vi "_FG_save_data.vi"(0 "enum":T1=enum."write", 2 "filenames (array)":string[](array[string]), 5 "entete":string, 7 "data in":variant, 9 "end":string, 11 "error in":errorcluster, 12 "array in line ?":bool, 13 "indexes to write":i32[](array[numeric])) -> (4 "path Array":path[](array[path]), 15 "error out":errorcluster)   [LabVIEW 2019]
uses:
  ae_save_data.ctl
  <userlib>/_OpenG.lib/array/array.llb/Index 1D Array Elements (Path)__ogtk.vi
  <vilib>/Utility/Data Type/NI_Data Type.lvlib
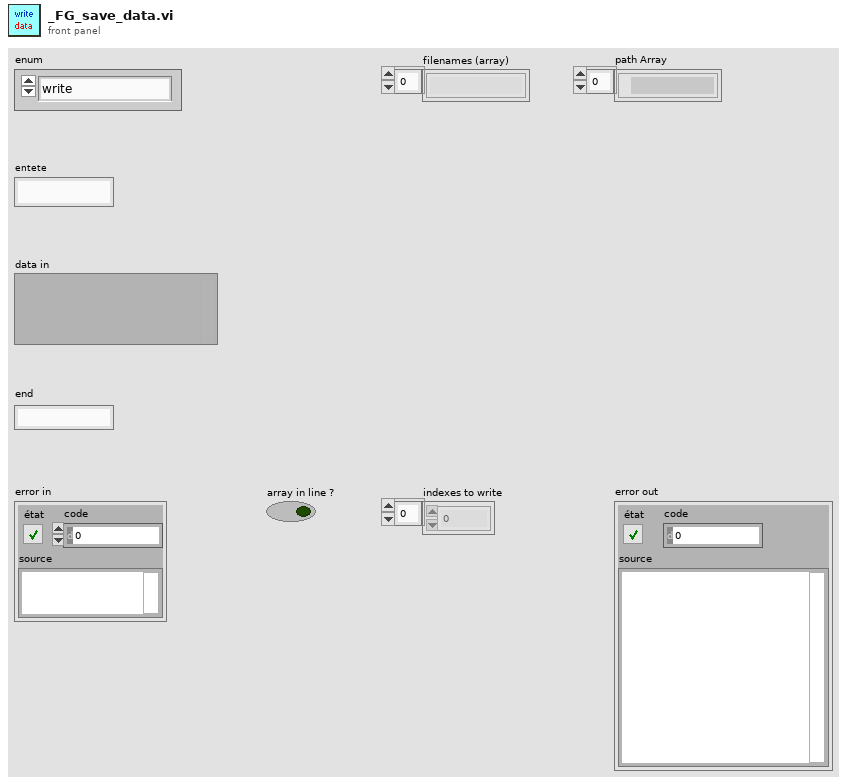
[diagram p1: front panel]
types:
  T1 = typedef "ae_save_data.ctl" = enum16{"create_file", "write", "time", "close_file", "read"}
  T2 = enum16{"open", "replace", "create", "open or create", "replace or create", "replace or create with confirmation"}
  T3 = typedef "NI_Data Type.lvlib/Data Type.ctl" = enum8{"Invalid Type", "Void", "I8", "I16", "I32", "I64", "U8", "U16", "U32", "U64", "Single Float", "Double Float", "Extended Float", "Single Complex", "Double Complex", "Extended Complex", "Enum U8", "Enum U16", "Enum U32", "Enum U64", "Single Float With Unit", "Double Float With Unit", "Extended Float With Unit", "Single Complex with Unit", "Double Complex with Unit", "Extended Complex with Unit", "Boolean", "String", "Path", "Picture", "Tag", "Array", "Cluster", "Variant", "LV Variant", "Waveform", "Timestamp", "Digital Waveform", "Digital Data", "ExpressData", "Refnum", "External Data", "VI", "Poly VI", "LabVIEW Class Instance", "Fixed Point", "Set Collection", "Map Collection"}
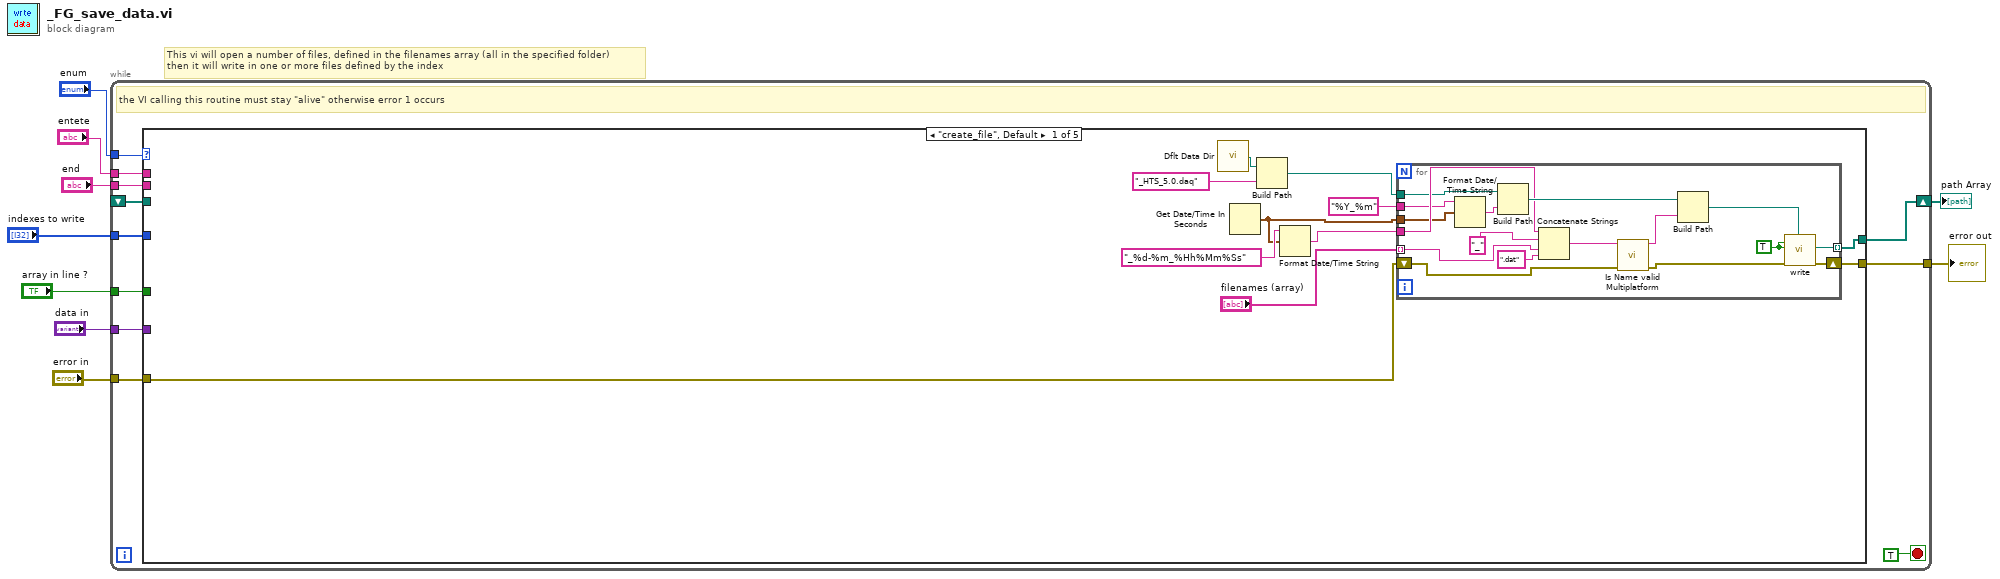
[diagram p0: block diagram]
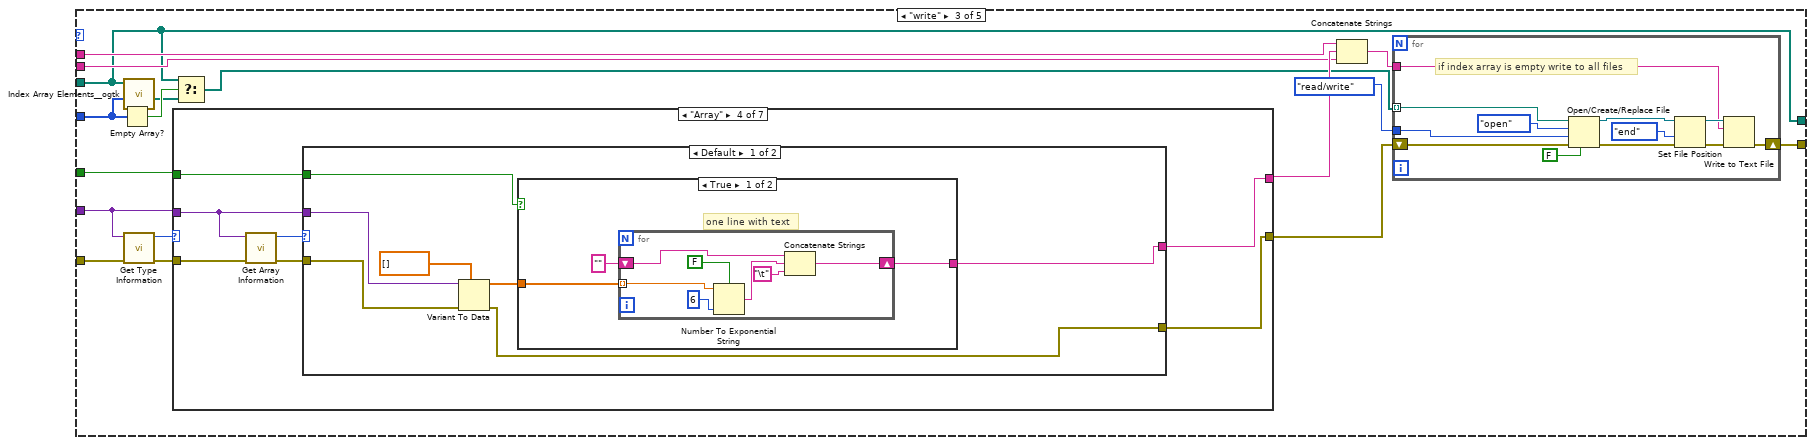
[diagram p3: hidden frame]
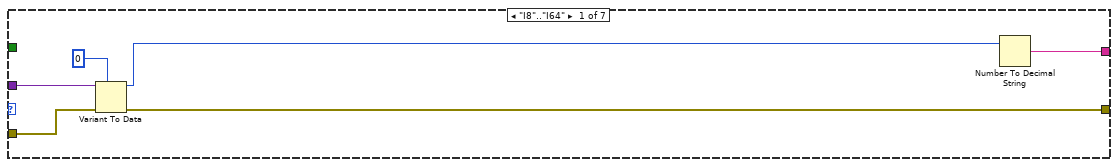
[diagram p4: hidden frame]
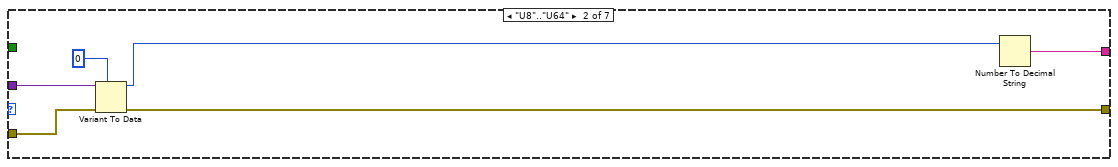
[diagram p5: hidden frame]
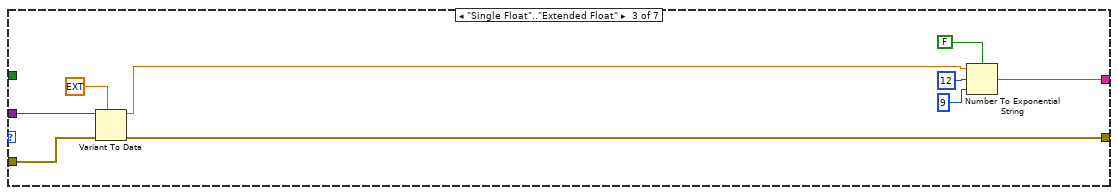
[diagram p6: hidden frame]
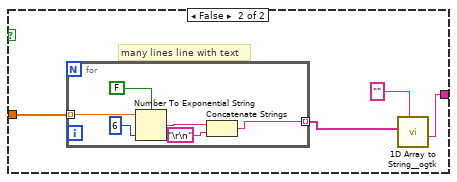
[diagram p7: hidden frame]
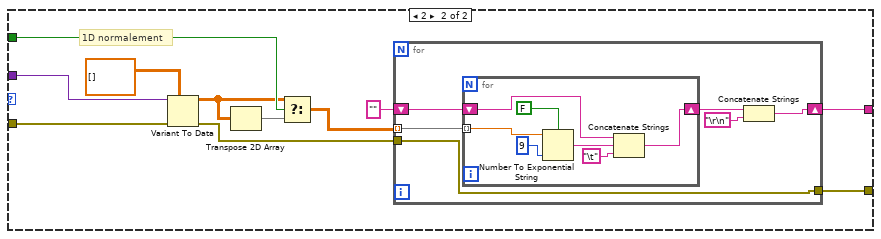
[diagram p8: hidden frame]
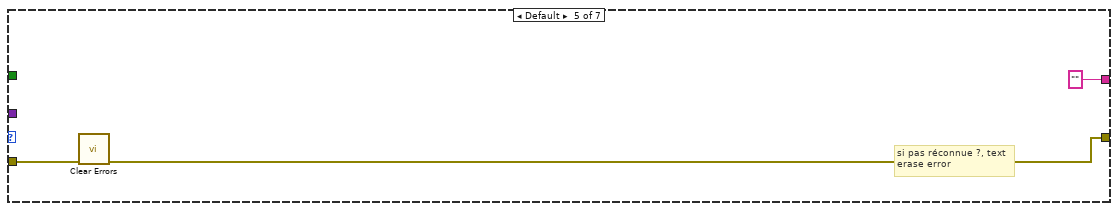
[diagram p9: hidden frame]
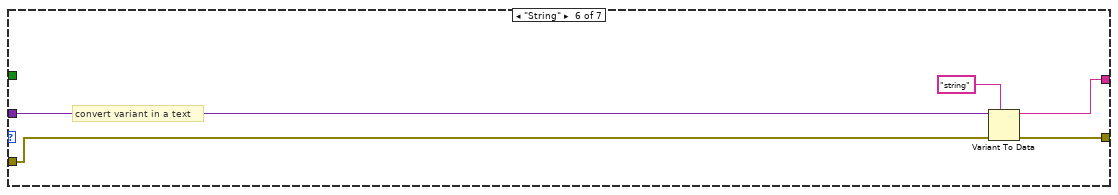
[diagram p10: hidden frame]
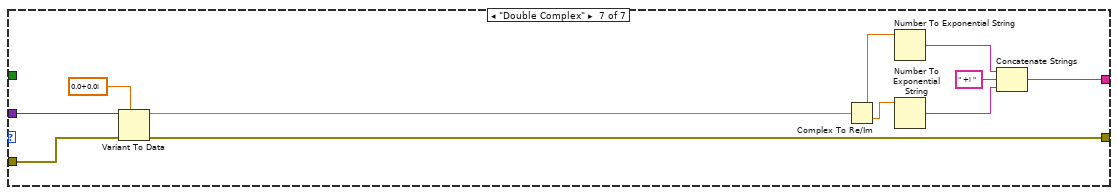
[diagram p11: hidden frame]
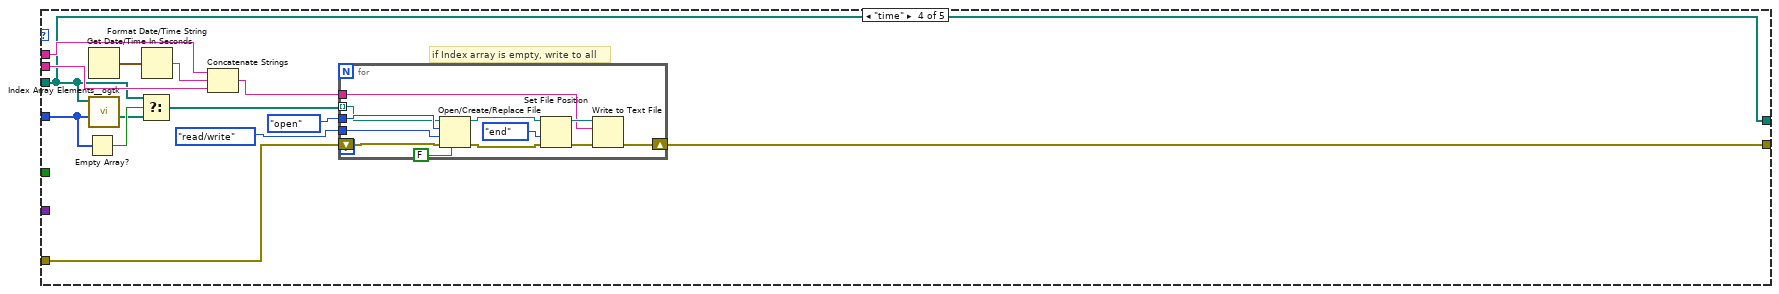
[diagram p12: hidden frame]
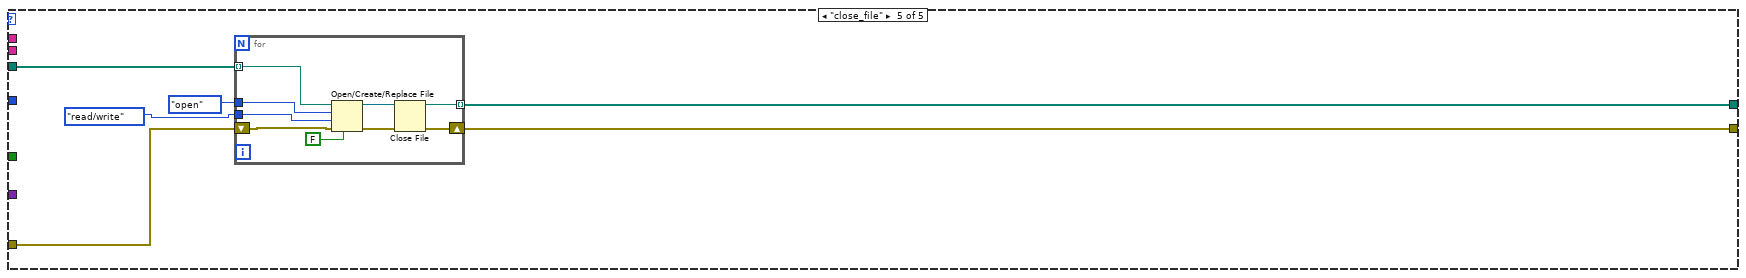
[diagram p13: hidden frame]
diagram:
  # "This vi will open a number of files, defined in the filenames array (all in the specified folder)\nthen it will write in one or more files defined by the index"
  n1 = while {
    tunnel: "enum" -> [w19]
    tunnel: "error in" -> [w18]
    tunnel: [w16] -> w7
    tunnel: "entete" -> [w17]
    shift-right: [w14] -> w1
    shift-left: _ -> [w15]
    tunnel: "array in line ?" -> [w13]
    tunnel: "data in" -> [w12]
    tunnel: "end" -> [w11]
    tunnel: "indexes to write" -> [w10]
    stop <- TRUE stop-if-true
    # "the VI calling this routine must stay \"alive\" otherwise error 1 occurs"
    n2 = case shown="\"create_file\", Default" w19 {
      tunnel: w18 -> [w29 w50 w64 w190 w209]
      tunnel: [w31 w50 w61 w187 w205] -> w16
      tunnel: w17 -> [_ _ w57 w186 _]
      tunnel: [w30 w49 w52 w180 w206] -> w14
      tunnel: w15 -> [_ w49 w52 w180 w204]
      tunnel: w13 -> [_ _ w65 _ _]
      tunnel: w12 -> [_ _ w58 _ _]
      tunnel: w11 -> [_ _ w56 w185 _]
      tunnel: w10 -> [_ _ w55 w182 _]
      frame "create_file", Default {
        n3 = call <vilib>:"Dflt Data Dir.vi"() -> ("App:Default Data Directory"=w24:path)
        n4 = Get Date/Time In Seconds() -> (seconds since 1Jan1904=w25:timestamp)
        n5 = Build Path(base path=w24, name or relative path="_HTS_5.0.daq") -> (appended path=w22:path)
        n6 = Format Date/Time String(time format string (%c)="_%d-%m_%Hh%Mm%Ss" ("format de l'heure (%c)"), seconds (now)=w25) -> (date/time string=w26:string)  [unwired: 1 in]
        n7 = for {
          tunnel: [w47] -> w30 mode=indexing
          shift-right: [w33] -> w31
          shift-left: w29 -> [w38]
          tunnel: "filenames (array)" -> [w36] mode=indexing
          tunnel: w26 -> [w40]
          tunnel: w25 -> [w39]
          tunnel: w22 -> [w35]
          tunnel: "%Y_%m" ("format de l'heure (%c)") -> [w32]
          w48 = TRUE ("Enable")
          n8 = Format Date/Time String(time format string (%c)=w32, seconds (now)=w39) -> (date/time string=w44:string)  [unwired: 1 in]
          n9 = Build Path(base path=w35, name or relative path=w44) -> (appended path=w45:path)
          n10 = Concatenate Strings(w40, "_" ("string"), w36, ".dat" ("string")) -> (w43:string)
          n11 = call "Is Name valid Multiplatform.vi"("error in (no error)"=w38, "filename"=w43) -> ("error out"=w34:errorcluster, "suggested filename"=w46:string)  [unwired: 5 in, 3 out]
          n12 = Build Path(base path=w45, name or relative path=w46) -> (appended path=w37:path)
          n13 = call "write"("Reset"=w48, "Enable"=w48, "error in (no error)"=w34, "Filename"=w37) -> ("Filename Out"=w47:path, "error out"=w33:errorcluster)  [unwired: 13 in, 1 out]
        }
      }
      frame "read" {
      }
      frame "write" {
        n14 = Empty Array?(array=w55) -> (empty?=w54:bool)
        n15 = call-poly <userlib>:"Index Array Elements__ogtk.vi"("indices"=w55, "array"=w52) -> ("elements"=w53:path[])  [unwired: 9 in]
        n16 = call <vilib>:"Get Type Information.vi"("error in (no error)"=w64, "variant"=w58) -> ("error out"=w66:errorcluster, "type"=w67:T3)  [unwired: 5 in, 3 out]
        n17 = case shown="\"Array\"" w67 {
          tunnel: w58 -> [w85 w91 w100 w104 _ w166 w177]
          tunnel: w66 -> [w84 w90 w99 w107 w160 w165 w175]
          tunnel: [w80 w86 w92 w102 "" ("Chaîne 2") w162 w167] -> w63
          tunnel: [w83 w89 w98 w101 w161 w164 w174] -> w60
          tunnel: w65 -> [_ _ _ w103 _ _ _]
          frame "I8".."I64" {
            n18 = Variant To Data(error in=w84, type=i64 0 ("r * e^(i*thêta)"), Variant=w85) -> (data=w81:i64, error out=w83:errorcluster)
            n19 = Number To Decimal String(number=w81) -> (decimal integer string=w80:string)  [unwired: 1 in]
          }
          frame "U8".."U64" {
            n20 = Variant To Data(error in=w90, type=u64 0 ("r * e^(i*thêta)"), Variant=w91) -> (data=w87:u64, error out=w89:errorcluster)
            n21 = Number To Decimal String(number=w87) -> (decimal integer string=w86:string)  [unwired: 1 in]
          }
          frame "Single Float".."Extended Float" {
            n22 = Variant To Data(error in=w99, type=ext 0.0 ("r * e^(i*thêta)"), Variant=w100) -> (data=w96:ext, error out=w98:errorcluster)
            n23 = Number To Exponential String(number=w96, precision (6)=i16 9 ("précision (6)"), 1:FALSE ("utiliser le séparateur décimal du système (V)"), 3:i16 12 ("largeur (-)")) -> (E-format string=w92:string)
          }
          frame "Array" {
            n24 = call <vilib>:"Get Array Information.vi"("error in (no error)"=w107, "variant"=w104) -> ("error out"=w105:errorcluster, "number of dimensions"=w106:i32)  [unwired: 6 in, 2 out]
            n25 = case shown="Default" w106 {
              tunnel: w105 -> [w113 w144]
              tunnel: w104 -> [w114 w145]
              tunnel: w103 -> [w110 w142]
              tunnel: [w108 w143] -> w102
              tunnel: [w111 w137] -> w101
              frame Default {
                n26 = Variant To Data(error in=w113, type=sgl[] [], Variant=w114) -> (data=w109:sgl[], error out=w111:errorcluster)
                n27 = case shown="True" w110 {
                  tunnel: w109 -> [w117 w128]
                  tunnel: [w116 w125] -> w108
                  frame True {
                    # "one line with text"
                    n28 = for {
                      tunnel: w117 -> [w124] mode=indexing
                      shift-right: [w123] -> w116
                      shift-left: "" -> [w119]
                      n29 = Number To Exponential String(number=w124, precision (6)=i16 6 ("précision (6)"), 1:FALSE ("utiliser le séparateur décimal du système (V)")) -> (E-format string=w120:string)  [unwired: 1 in]
                      n30 = Concatenate Strings(w119, w120, "\t") -> (w123:string)
                    }
                  }
                  frame False {
                    # "many lines line with text"
                    n31 = for {
                      tunnel: w128 -> [w134] mode=indexing
                      tunnel: [w130] -> w127 mode=indexing
                      n32 = Number To Exponential String(number=w134, precision (6)=i16 6 ("précision (6)"), 1:FALSE ("utiliser le séparateur décimal du système (V)")) -> (E-format string=w131:string)  [unwired: 1 in]
                      n33 = Concatenate Strings(w131, "\r\n") -> (w130:string)
                    }
                    n34 = call <userlib>:"1D Array to String__ogtk.vi"("delimiter (Tab)"="", "Array of Strings"=w127) -> ("delimited string"=w125:string)  [unwired: 9 in]
                  }
                }
              }
              frame 2 {
                # "1D normalement"
                n35 = Variant To Data(error in=w144, type=sgl[][] [] ("tableau ajouté"), Variant=w145) -> (data=w140:sgl[][], error out=w136:errorcluster)
                n36 = Transpose 2D Array(2D array=w140) -> (transposed array=w139:sgl[][])
                n37 = Select(t=w140, s=w142, f=w139) -> (s? t:f=w138:sgl[][])
                n38 = for {
                  tunnel: w138 -> [w151] mode=indexing
                  shift-right: [w147] -> w143
                  shift-left: "" -> [w150]
                  tunnel: [w146] -> w137
                  tunnel: w136 -> [w146]
                  n39 = for {
                    tunnel: w151 -> [w158] mode=indexing
                    shift-right: [w156] -> w148
                    shift-left: w150 -> [w155]
                    n40 = Number To Exponential String(number=w158, precision (6)=i16 9 ("précision (6)"), 1:FALSE ("utiliser le séparateur décimal du système (V)")) -> (E-format string=w157:string)  [unwired: 1 in]
                    n41 = Concatenate Strings(w155, w157, "\t") -> (w156:string)
                  }
                  n42 = Concatenate Strings(w148, "\r\n") -> (w147:string)
                }
              }
            }
          }
          frame Default {
            # "si pas réconnue ?, text\nerase error"
            n43 = call <vilib>:"Clear Errors.vi"("error in (no error)"=w160) -> ("error out"=w161:errorcluster)  [unwired: 5 in, 1 out]
          }
          frame "String" {
            # "convert variant in a text"
            n44 = Variant To Data(error in=w165, type="string" ("Chaîne 2"), Variant=w166) -> (data=w162:string, error out=w164:errorcluster)
          }
          frame "Double Complex" {
            n45 = Variant To Data(error in=w175, type=cdb 0.0+0.0i, Variant=w177) -> (data=w173:cdb, error out=w174:errorcluster)
            n46 = Complex To Re/Im(x + iy=w173) -> (x=w172:dbl, y=w171:dbl)
            n47 = Number To Exponential String(number=w172) -> (E-format string=w170:string)  [unwired: 3 in]
            n48 = Number To Exponential String(number=w171) -> (E-format string=w169:string)  [unwired: 3 in]
            n49 = Concatenate Strings(w170, " +i " ("chaîne"), w169) -> (w167:string)
          }
        }
        n50 = Select(t=w52, s=w54, f=w53) -> (s? t:f=w51:path[])
        n51 = Concatenate Strings(w57, w63, w56) -> (w59:string)
        n52 = for {
          tunnel: enum16{"read/write", "read-only", "write-only"}."read/write" ("accès (0 : read/write)") -> [w73]
          tunnel: w59 -> [w69]
          shift-right: [w71] -> w61
          shift-left: w60 -> [w70]
          tunnel: w51 -> [w68] mode=indexing
          # "if index array is empty write to all files"
          n53 = Open/Create/Replace File(file path (use dialog)=w68, error in=w70, operation (0:open)=T2."open" ("opération (0 : open)"), access (0:read/write)=w73, disable buffering (F)=FALSE ("désactiver la bufférisation (F)")) -> (refnum out=w79:refnum<file>, error out=w75:errorcluster)  [unwired: 1 in, 1 out]
          n54 = Set File Position(refnum=w79, from (0:start)=enum16{"start", "end", "current"}."end" ("à partir de (0 : start)"), error in=w75) -> (refnum out=w77:refnum<file>, error out=w74:errorcluster)  [unwired: 1 in]
          n55 = Write to Text File(file (use dialog)=w77, text=w69, error in=w74) -> (error out=w71:errorcluster)  [unwired: 1 in, 2 out]
        }
      }
      frame "time" {
        # "if Index array is empty, write to all"
        n56 = Empty Array?(array=w182) -> (empty?=w181:bool)
        n57 = Get Date/Time In Seconds() -> (seconds since 1Jan1904=w191:timestamp)
        n58 = call-poly <userlib>:"Index Array Elements__ogtk.vi"("indices"=w182, "array"=w180) -> ("elements"=w179:path[])  [unwired: 9 in]
        n59 = Select(t=w180, s=w181, f=w179) -> (s? t:f=w178:path[])
        n60 = Format Date/Time String(seconds (now)=w191) -> (date/time string=w184:string)  [unwired: 2 in]
        n61 = Concatenate Strings(w186, w184, w185) -> (w183:string)
        n62 = for {
          tunnel: enum16{"read/write", "read-only", "write-only"}."read/write" ("accès (0 : read/write)") -> [w196]
          tunnel: T2."open" ("opération (0 : open)") -> [w195]
          tunnel: w183 -> [w193]
          shift-right: [w194] -> w187
          shift-left: w190 -> [w203]
          tunnel: w178 -> [w192] mode=indexing
          n63 = Open/Create/Replace File(file path (use dialog)=w192, error in=w203, operation (0:open)=w195, access (0:read/write)=w196, disable buffering (F)=FALSE ("désactiver la bufférisation (F)")) -> (refnum out=w202:refnum<file>, error out=w198:errorcluster)  [unwired: 1 in, 1 out]
          n64 = Set File Position(refnum=w202, from (0:start)=enum16{"start", "end", "current"}."end" ("à partir de (0 : start)"), error in=w198) -> (refnum out=w200:refnum<file>, error out=w197:errorcluster)  [unwired: 1 in]
          n65 = Write to Text File(file (use dialog)=w200, text=w193, error in=w197) -> (error out=w194:errorcluster)  [unwired: 1 in, 2 out]
        }
      }
      frame "close_file" {
        n66 = for {
          tunnel: enum16{"read/write", "read-only", "write-only"}."read/write" ("accès (0 : read/write)") -> [w216]
          tunnel: T2."open" ("opération (0 : open)") -> [w215]
          tunnel: [w214] -> w206 mode=indexing
          tunnel: w204 -> [w212] mode=indexing
          shift-right: [w213] -> w205
          shift-left: w209 -> [w218]
          n67 = Open/Create/Replace File(file path (use dialog)=w212, error in=w218, operation (0:open)=w215, access (0:read/write)=w216, disable buffering (F)=FALSE ("désactiver la bufférisation (F)")) -> (refnum out=w211:refnum<file>, error out=w210:errorcluster)  [unwired: 1 in, 1 out]
          n68 = Close File(refnum=w211, error in=w210) -> (path=w214:path, error out=w213:errorcluster)
        }
      }
    }
  }
  "error out" <- w7
  "path Array" <- w1
